vi "Find Added Highlight in Parenthesis.vi"(11 "Test Case In":refnum<class "Find Highlights Test.lvclass">) -> (0 "error out":errorcluster, 3 "Test Case Out":refnum<class "Find Highlights Test.lvclass">)   [LabVIEW 2020, in "Find Highlights Test.lvclass"]
uses:
  Find Highlights Test.lvclass
  usr/local/natinst/LabVIEW-2026-64/vi.lib/Astemes/LUnit/Test Case.lvclass
  <vilib>/Astemes/LUnit/Test Case.lvclass/Test Case.ctl
  4993e8ee-a06a-463a-9684-69129f64d5ce.vi
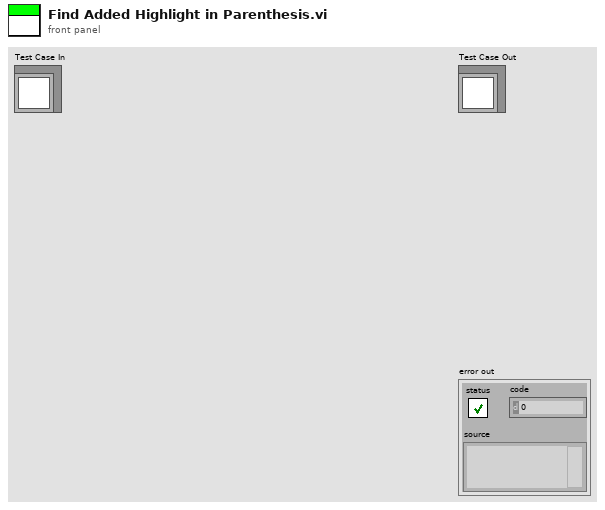
[diagram p1: front panel]
types:
  T1 = cluster{"Selection Start":u32, "Selection End":u32, "Type":enum16{"added", "missing"}}
  T2 = cluster{"Selection Start":u32, "Selection End":u32, "Type":enum16{"added", "missing"}}[]
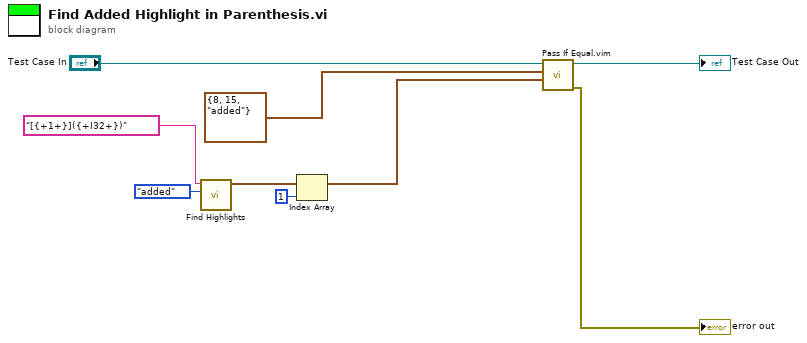
[diagram p0: block diagram]
diagram:
  n1 = call "Find Highlights.vi"("Type"=enum16{"added", "missing"}."added", "String"="[{+1+}]({+I32+})" ("Reference")) -> ("Sections"=w4:T2)  [unwired: 9 in]
  n2 = Index Array(array=w4, index=1) -> (element=w2:T1)
  n3 = call "Pass If Equal.vim"("Actual"=w2, "Expected"=T1 {"Selection Start"=8, "Selection End"=15, "Type"=enum."added"}, "LUnit Test Case In"="Test Case In") -> ("error out"=→"error out":errorcluster, "LUnit Test Case Out"=→"Test Case Out":refnum<class "Find Highlights Test.lvclass">)  [unwired: 7 in]
